vi "IOR4 Relay Control MAIN.vi"(8 "error in (no error)":errorcluster, 10 "#Writes per cmd":enum16{"1", "2", "3", "4", "5"}(ring)=enum."2", 11 "Relay Control Sequencer":T1(array[ring])) -> (0 "error out":errorcluster)   [LabVIEW 2020, in "DLP Design Modules Driver.lvlib"]
doc: "Developed By: J Branch\nLast Update: 10/9/2022\n\nDescription: Allows user control of the DLP IOR4 relay module through LabVIEW. This relay module is a relatively simple to use programatically contolled USB relay module with 4 SPDT 2A latching relays.\n\nSee the datasheet from DLP Design to view more about the device description."
uses:
  DLP Design Modules Driver.lvlib
panel:
  in  "Tab Control":enum32{"User", "Back Params"}(tab)
  out "UserMsg":string="Specify relay actions to be performed using the Relay Control Sequencer prior to running the program.\n\nThe #Writes per cmd determines how many times each relay control command is sent over the COM port connection between LabVIEW and the IOR4 device.  More writes reduces the chances of error caused by the device failing to respond to a sent command, but will make the program run slower."
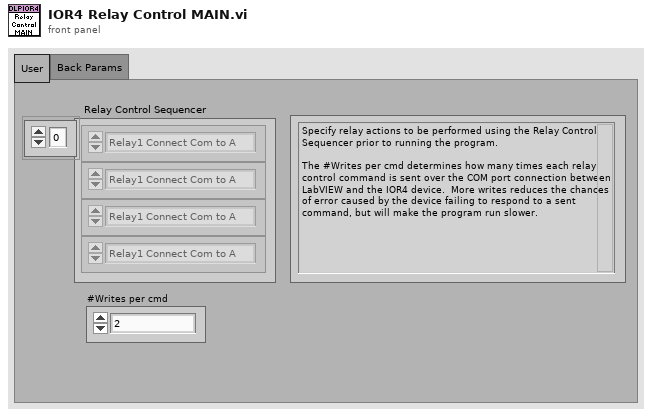
[diagram p1: front panel]
types:
  T1 = enum16{"Relay1 Connect Com to A", "Relay1 Connect Com to B", "Relay2 Connect Com to A", "Relay2 Connect Com to B", "Relay3 Connect Com to A", "Relay3 Connect Com to B", "Relay4 Connect Com to A", "Relay4 Connect Com to B"}[]
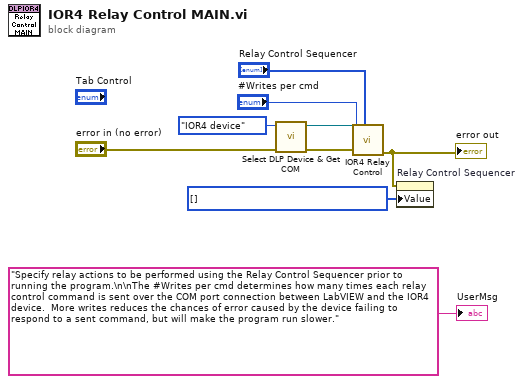
[diagram p0: block diagram]
diagram:
  w1 = T1 [] items=["Relay1 Connect Com to A", "Relay1 Connect Com to B", "Relay2 Connect Com to A", "Relay2 Connect Com to B", "Relay3 Connect Com to A", "Relay3 Connect Com to B", "Relay4 Connect Com to A", "Relay4 Connect Com to B"] ("Relay Control Sequencer")
  n1 = call "Select DLP Device & Get COM.vi"("error in (no error)"="error in (no error)", "Device Type Selection"=enum16{"IOR4 device", "IO20 device"}."IOR4 device") -> ("error out"=w7:errorcluster, "Selected COM"=w8:refnum<visa-resource-name>)  [unwired: 7 in, 1 out]
  n2 = call "IOR4 Relay Control .vi"("Relay Control Sequence"="Relay Control Sequencer", "error in (no error)"=w7, "#Writes per cmd"="#Writes per cmd", "Relay ComPort"=w8) -> ("error out"=w2:errorcluster)  [unwired: 7 in]
  "error out" <- w2
  n3 = property on="Relay Control Sequencer" class="Arr (strict)"(error in=w2, "Value"=w1) -> ()  [unwired: 1 in, 2 out]
  "UserMsg" <- "Specify relay actions to be performed using the Relay Control Sequencer prior to running the program.\n\nThe #Writes per cmd determines how many times each relay control command is sent over the COM port connection between LabVIEW and the IOR4 device.  More writes reduces the chances of error caused by the device failing to respond to a sent command, but will make the program run slower." ("UserMsg")
